vi "Example.api.vi"(10 "Baud Rate":u32(ring)=57600 items=["75"=75, "110"=110, "134"=134, "150"=150, "300"=300, "600"=600, "1200"=1200, "1800"=1800, "2400"=2400, "4800"=4800, "7200"=7200, "9600"=9600, "14400"=14400, "19200"=19200, "28800"=28800, "38400"=38400, "56000"=56000, "57600"=57600, "115200"=115200, "128000"=128000, "230400"=230400], 11 "Comport":refnum<visa-resource-name>="COM20") -> (0 "error out":errorcluster)   [LabVIEW 2020]
doc: "Initializes the library with a serial comport as the transport method"
uses:
  FirmataClient/Controls/FirmataPinCapabilitiesAndAnalogMapping.ctl
  FirmataClient/Controls/FirmataPinCapability.ctl
  FirmataClient/Controls/FirmataPinModes.ctl
  FirmataClient/FirmataClient.lvlib
panel:
  in  "Stop":bool
  in  "Tab Control":enum32{"Connection", "API"}(tab)
  in  "Connection Details":enum32{"Serial Communication"}(tab)
  out "Firmata Firmware Version":string
  out "Firmata Firmware Name":string
  in  "Query Capabilities?":bool
  in  "Button":bool
  out "Board Capabilities":map{i32, T1}(c390)
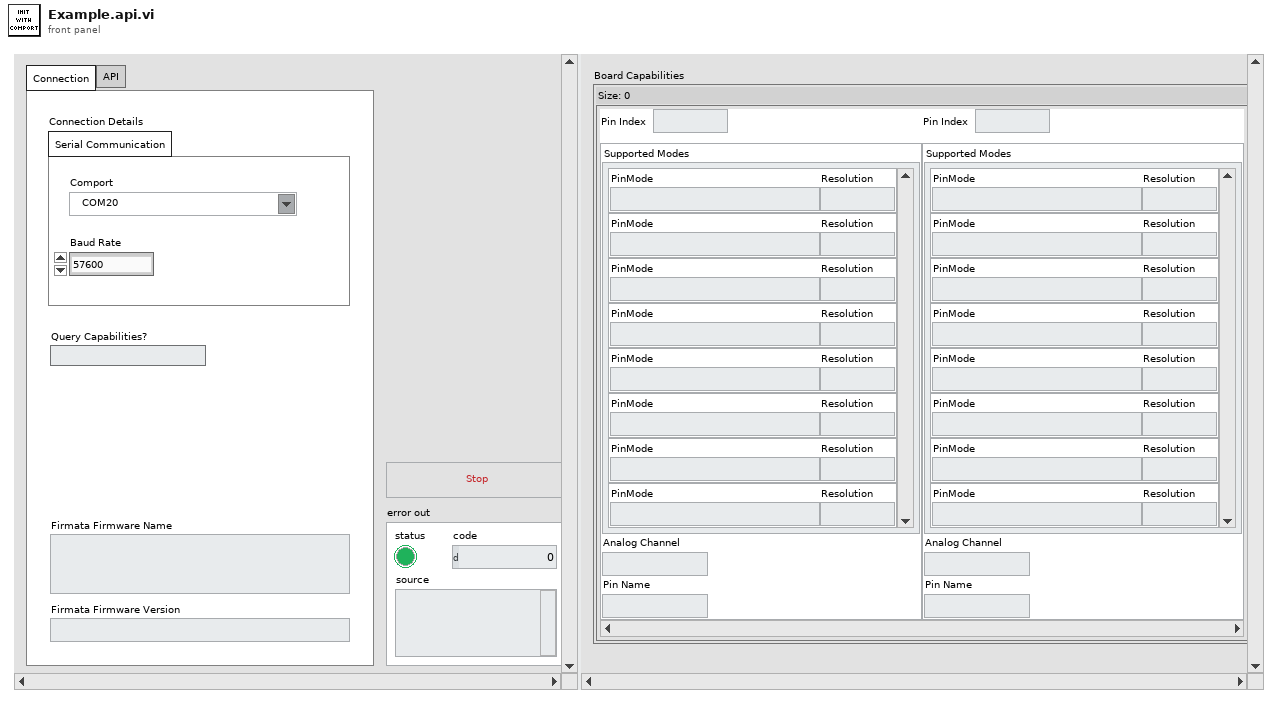
[diagram p1: front panel]
types:
  T1 = typedef "FirmataClient.lvlib/FirmataPinCapabilitiesAndAnalogMapping.ctl" = cluster{"Supported Modes":T2[], "Analog Channel":u8, "Pin Name":string}
  T2 = typedef "FirmataClient.lvlib/FirmataPinCapability.ctl" = cluster{"PinMode":T3, "Resolution":u8}
  T3 = typedef "FirmataClient.lvlib/FirmataPinModes.ctl" = enum16{"DigitalInput", "DigitalOutput", "AnalogInput", "PWM", "Servo", "Shift", "I2C", "OneWire", "Stepper", "Encoder", "Serial", "InputPullup", "Extended.SPI", "Extended.Sonar", "Extended.Tone", "Extended.DHT"}
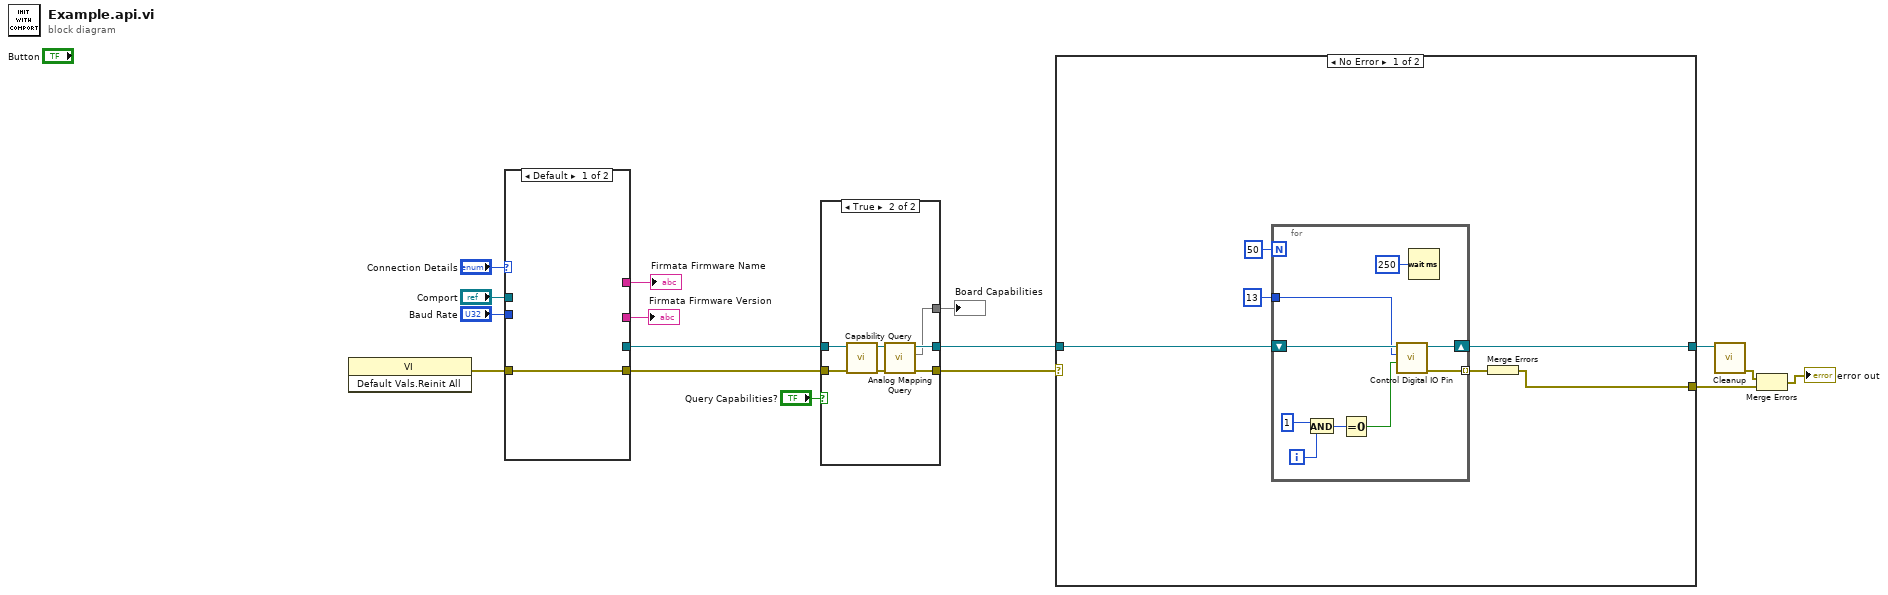
[diagram p0: block diagram]
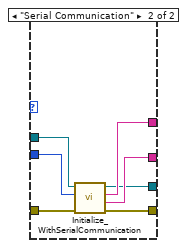
[diagram p3: hidden frame]
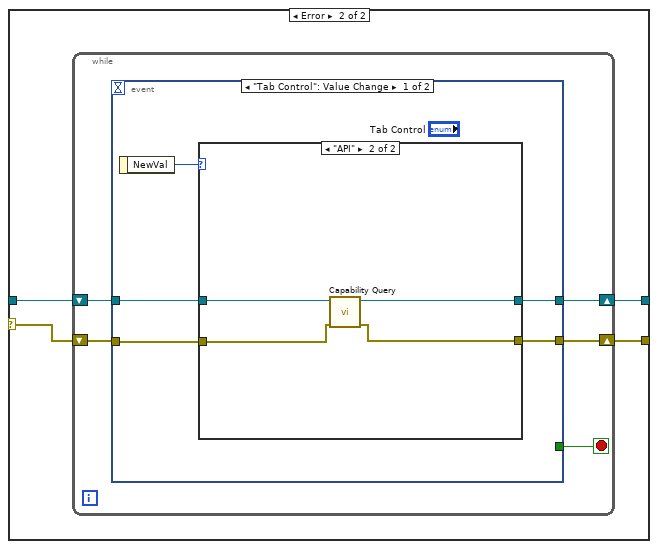
[diagram p4: hidden frame]
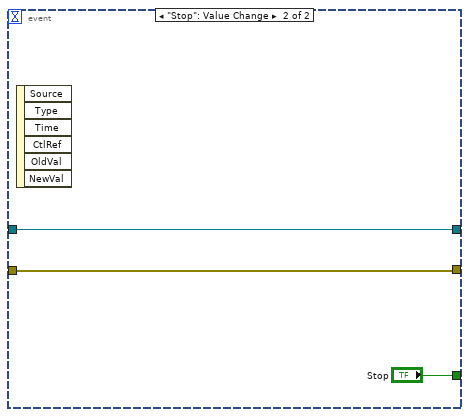
[diagram p6: hidden frame]
diagram:
  n1 = invoke class="VI" method="Default Vals.Reinit All"() -> (error out=w14:errorcluster)  [unwired: 3 in, 2 out]
  n2 = case shown="Default" "Connection Details" {
    tunnel: w14 -> [w17 w24]
    tunnel: "Baud Rate" -> [_ w23]
    tunnel: "Comport" -> [_ w22]
    tunnel: [_ w21] -> w11
    tunnel: [_ w20] -> w10
    tunnel: [_ w19] -> w7
    tunnel: [w17 w18] -> w6
    frame Default {
    }
    frame "Serial Communication" {
      n3 = call "Initialize_WithSerialCommunication.vi"("error in"=w24, "Baud Rate"=w23, "Comport"=w22) -> ("error out"=w18:errorcluster, "FirmataFirmwareVersion"=w20:string, "FirmataFirmwareName"=w21:string, "Refnum Out"=w19:refnum<vi>)  [unwired: 4 in, 1 out]
    }
  }
  "Firmata Firmware Name" <- w11
  "Firmata Firmware Version" <- w10
  n4 = case shown="True" "Query Capabilities?" {
    tunnel: w7 -> [w26 w33]
    tunnel: w6 -> [w25 w32]
    tunnel: [w26 w29] -> w5
    tunnel: [w25 w28] -> w4
    tunnel: [_ w27] -> w2
    frame False {
    }
    frame True {
      n5 = call "Capability Query.vi"("error in (no error)"=w32, "Refnum In"=w33) -> ("error out"=w30:errorcluster, "Refnum Out"=w31:refnum<vi>)  [unwired: 7 in, 1 out]
      n6 = call "Analog Mapping Query.vi"("error in (no error)"=w30, "Refnum In"=w31) -> ("error out"=w28:errorcluster, "Board Capabilities"=w27:map{i32, T1}, "Refnum Out"=w29:refnum<vi>)  [unwired: 7 in]
    }
  }
  "Board Capabilities" <- w2
  n7 = case shown="No Error" w4 {
    selector: w4 -> [_ w49]
    tunnel: [w34 w52] -> w9
    tunnel: [w38 w51] -> w8
    tunnel: w5 -> [w39 w50]
    frame No Error {
      n8 = for {
        N: 50 -> [_]
        tunnel: u8 13 ("Port Index") -> [w46]
        shift-right: [w47] -> w38
        shift-left: w39 -> [w48]
        tunnel: [w40] -> w35 mode=indexing
        i -> [w44]
        n9 = And(x=1, y=w44) -> (x .and. y?=w42:i32)
        n10 = Equal To 0?(x=w42) -> (x = 0?=w41:bool)
        n11 = call "Control Digital IO Pin.vi"("Pin Value"=w41, "Pin Index"=w46, "Refnum In"=w48) -> ("error out"=w40:errorcluster, "Refnum Out"=w47:refnum<vi>)  [unwired: 5 in, 2 out]
        n12 = Wait (ms)(milliseconds to wait=u32 250) -> ()  [unwired: 1 out]
      }
      n13 = Merge Errors(w35) -> (w34:errorcluster)
    }
    frame Error {
      n14 = while {
        shift-right: [w56] -> w51
        shift-left: w50 -> [w55]
        shift-right: [w57] -> w52
        shift-left: w49 -> [w54]
        stop <- w53 stop-if-true
        n15 = event shown="[0] \"Tab Control\": Value Change" {
          selector: _ -> [_ _]
          dyn-events: _ -> [_ _]
          timeout: _ -> [_ _]
          tunnel: [w62 w69] -> w57
          tunnel: w54 -> [w61 w69]
          tunnel: [w60 w70] -> w56
          tunnel: w55 -> [w59 w70]
          tunnel: [_ "Stop"] -> w53
          event "Tab Control": Value Change {
            n16 = event-data() -> ("NewVal"=w58:enum32{"Connection", "API"})  [unwired: 1 in]
            n17 = case shown="\"API\"" w58 {
              tunnel: [w63 w65] -> w62
              tunnel: w61 -> [w63 w66]
              tunnel: [w64 w67] -> w60
              tunnel: w59 -> [w64 w68]
              frame "Connection", Default {
              }
              frame "API" {
                n18 = call "Capability Query.vi"("error in (no error)"=w66, "Refnum In"=w68) -> ("error out"=w65:errorcluster, "Refnum Out"=w67:refnum<vi>)  [unwired: 7 in, 1 out]
              }
            }
          }
          event "Stop": Value Change {
            n19 = event-data() -> ()  [unwired: 1 in, 6 out]
          }
        }
      }
    }
  }
  n20 = call "Cleanup.vi"("Refnum In"=w8) -> ("error out"=w16:errorcluster)  [unwired: 10 in]
  n21 = Merge Errors(w16, w9) -> (→"error out":errorcluster)
